vi "Demo.vi"() -> ()   [LabVIEW 2018]
uses:
  api/Log Levels.ctl
  api/Failure Information.ctl
  api/Log Record.ctl
  api/logger_class/Internal Log Levels.ctl
  api/extension/filter_interface/Match Behavior.ctl
  5758470c-db3e-42ca-811c-825e9724b0d9.vi
  30f214a0-5d11-42b7-bf48-9498a62074b5.vi
  4d4d1e0d-ca84-4252-a363-7338c056865d.vi
  e9fdd159-732b-4b71-b39a-13da20540399.vi
  514e4c3d-4430-404b-bd65-5c4555decd7a.vi
  f7cffa30-522c-4f2e-8b3f-df899d765069.vi
  6bf7c309-aeaa-44f2-9fe0-d02c6e1e6f2a.vi
  b04b80c8-7d4a-4373-a7ed-4e6fc68618ba.vi
  82079a54-0ade-4b6d-97e0-3412ec680245.vi
  28c04e52-e175-4a95-b6fe-3645044e5316.vi
  f0baf2eb-a7d9-4d62-b153-bba25fce558d.vi
  f6dcc986-d3e7-4001-b7d2-0cb11a3872ca.vi
  8dbb979e-3c8b-43bd-9788-6e6dcdfca317.vi
  5758470c-db3e-42ca-811c-825e9724b0d9.vi/caf2d4a3-5a7b-40e1-b7b0-74b52901b9f9.vi
  30f214a0-5d11-42b7-bf48-9498a62074b5.vi/bf655d3c-1ce4-400f-a78f-0f3f0191886e.vi
  api/Mark Error.vi
  4d4d1e0d-ca84-4252-a363-7338c056865d.vi/bf655d3c-1ce4-400f-a78f-0f3f0191886e.vi
  e9fdd159-732b-4b71-b39a-13da20540399.vi/ba94d47b-0e30-4c32-b8ff-86d609cd95a5.vi
  514e4c3d-4430-404b-bd65-5c4555decd7a.vi/ba94d47b-0e30-4c32-b8ff-86d609cd95a5.vi
  f7cffa30-522c-4f2e-8b3f-df899d765069.vi/de1063af-56d8-4a46-86b0-d7db6137800f.vi
  6bf7c309-aeaa-44f2-9fe0-d02c6e1e6f2a.vi/de1063af-56d8-4a46-86b0-d7db6137800f.vi
  b04b80c8-7d4a-4373-a7ed-4e6fc68618ba.vi/6f202c45-f0ca-42f4-9f63-a87d9fe0c32d.vi
  82079a54-0ade-4b6d-97e0-3412ec680245.vi/73f0ec31-6bdf-4568-9d3b-fef50ac01b30.vi
  28c04e52-e175-4a95-b6fe-3645044e5316.vi/0a1ee2ab-da6d-4243-8cf3-8125e611a602.vi
  5758470c-db3e-42ca-811c-825e9724b0d9.vi/caf2d4a3-5a7b-40e1-b7b0-74b52901b9f9.vi/0a1ee2ab-da6d-4243-8cf3-8125e611a602.vi
  api/configuration/scopes/basic_scope/Basic.lvclass
  C:/Users/Colin/Documents/software_projects/labview/glog/src/api/extension/scope_interface/Scope.lvclass
  api/configuration/formatters/format_string_formatter/Format String.lvclass
  C:/Users/Colin/Documents/software_projects/labview/glog/src/api/extension/formatter_interface/Formatter.lvclass
  api/configuration/handlers/string_handler/String Handler.lvclass
  C:/Users/Colin/Documents/software_projects/labview/glog/src/api/extension/formatting_handler_interface/Formatting Handler.lvclass
  api/configuration/handlers/file_handler/File Handler.lvclass
  api/configuration/scopes/basic_scope/New (Element).vi
  registry/Log.vi
  <vilib>/Utility/error.llb/Error Cluster From Error Code.vi
  registry/Enable All.vi
  registry/Disable All.vi
  <vilib>/ErrorRing/Error Ring.xnode
  api/GLog.lvlib
panel:
  in  "format string":T1(ring)
  in  "include descendants?":bool caption="Include Descendants?"
  in  "match behavior":T2
  in  "scope":enum16{"Demo", "SubVI", "SubSubVI"}(ring)
  in  "call tree loop":bool caption="Enable Loop"
  in  "error loop":bool caption="Enable Loop"
  in  "basic loop":bool caption="Enable Loop"
  out "log directory":path
  in  "log delay [ms]":i32=100
  in  "log files":i32(listbox)
  in  "error":bool
  in  "warn":bool
  out "failures info":T3[](array[typedef]) {"Log Record"."timestamp" format="%<%x %.3X>T"}
  out "error out":errorcluster
  in  "set lvl all":bool
  in  "disable all":bool
  in  "enable all":bool
  in  "set lvl":bool
  in  "log level":T6
  in  "Loggers":i32(listbox)
  in  "Quit":bool
  out "string logs":string
  in  "disable":bool
  in  "enable":bool
  # "State Control"
  # "Log Level Control"
  # "Speed"
  # "Generic Logging"
  # "Errors/Warnings"
  # "SubVIs"
  # "%^<%Y-%m-%dT%H:%M:%S%3uZ>T | %8L | %M"
  # "%<%a, %b %d, %Y | %I:%M %p>T | %8L | %M"
  # "%<%I:%M:%S %p>T | %8L | %M"
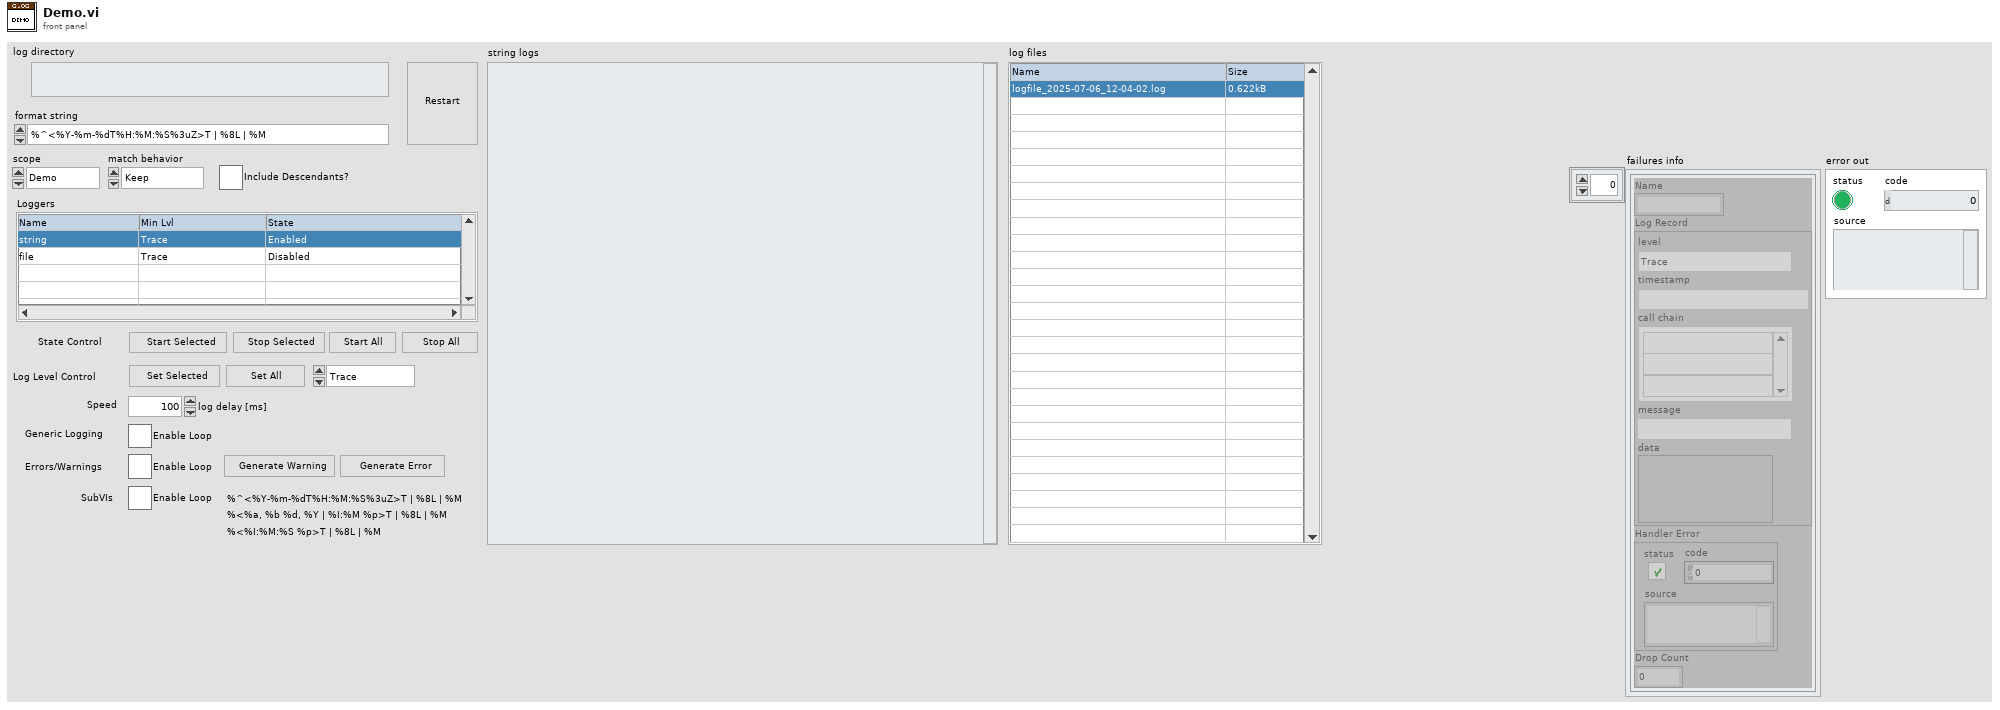
[diagram p1: front panel]
types:
  T1 = enum16{"%^<%Y-%m-%dT%H:%M:%S%3uZ>T | %8L | %M", "%<%a, %b %d, %Y | %I:%M %p>T | %8L | %M", "%<%I:%M:%S %p>T | %8L | %M", "%-30M | %C"}
  T2 = typedef "GLog.lvlib/Match Behavior.ctl" = enum16{"Keep", "Discard"}
  T3 = typedef "GLog.lvlib/Failure Information.ctl" = cluster{"Name":string, "Log Record":T4, "Handler Error":errorcluster, "Drop Count":u32}
  T4 = typedef "GLog.lvlib/Log Record.ctl" = cluster{"level":T5, "timestamp":timestamp, "call chain":string[], "message":string, "data":variant}
  T5 = typedef "GLog.lvlib/Internal Log Levels.ctl" = enum16{"Trace", "Debug", "Info", "Warning", "Error", "Critical", "Internal"}
  T6 = typedef "GLog.lvlib/Log Levels.ctl" = enum16{"Trace", "Debug", "Info", "Warning", "Error", "Critical"}
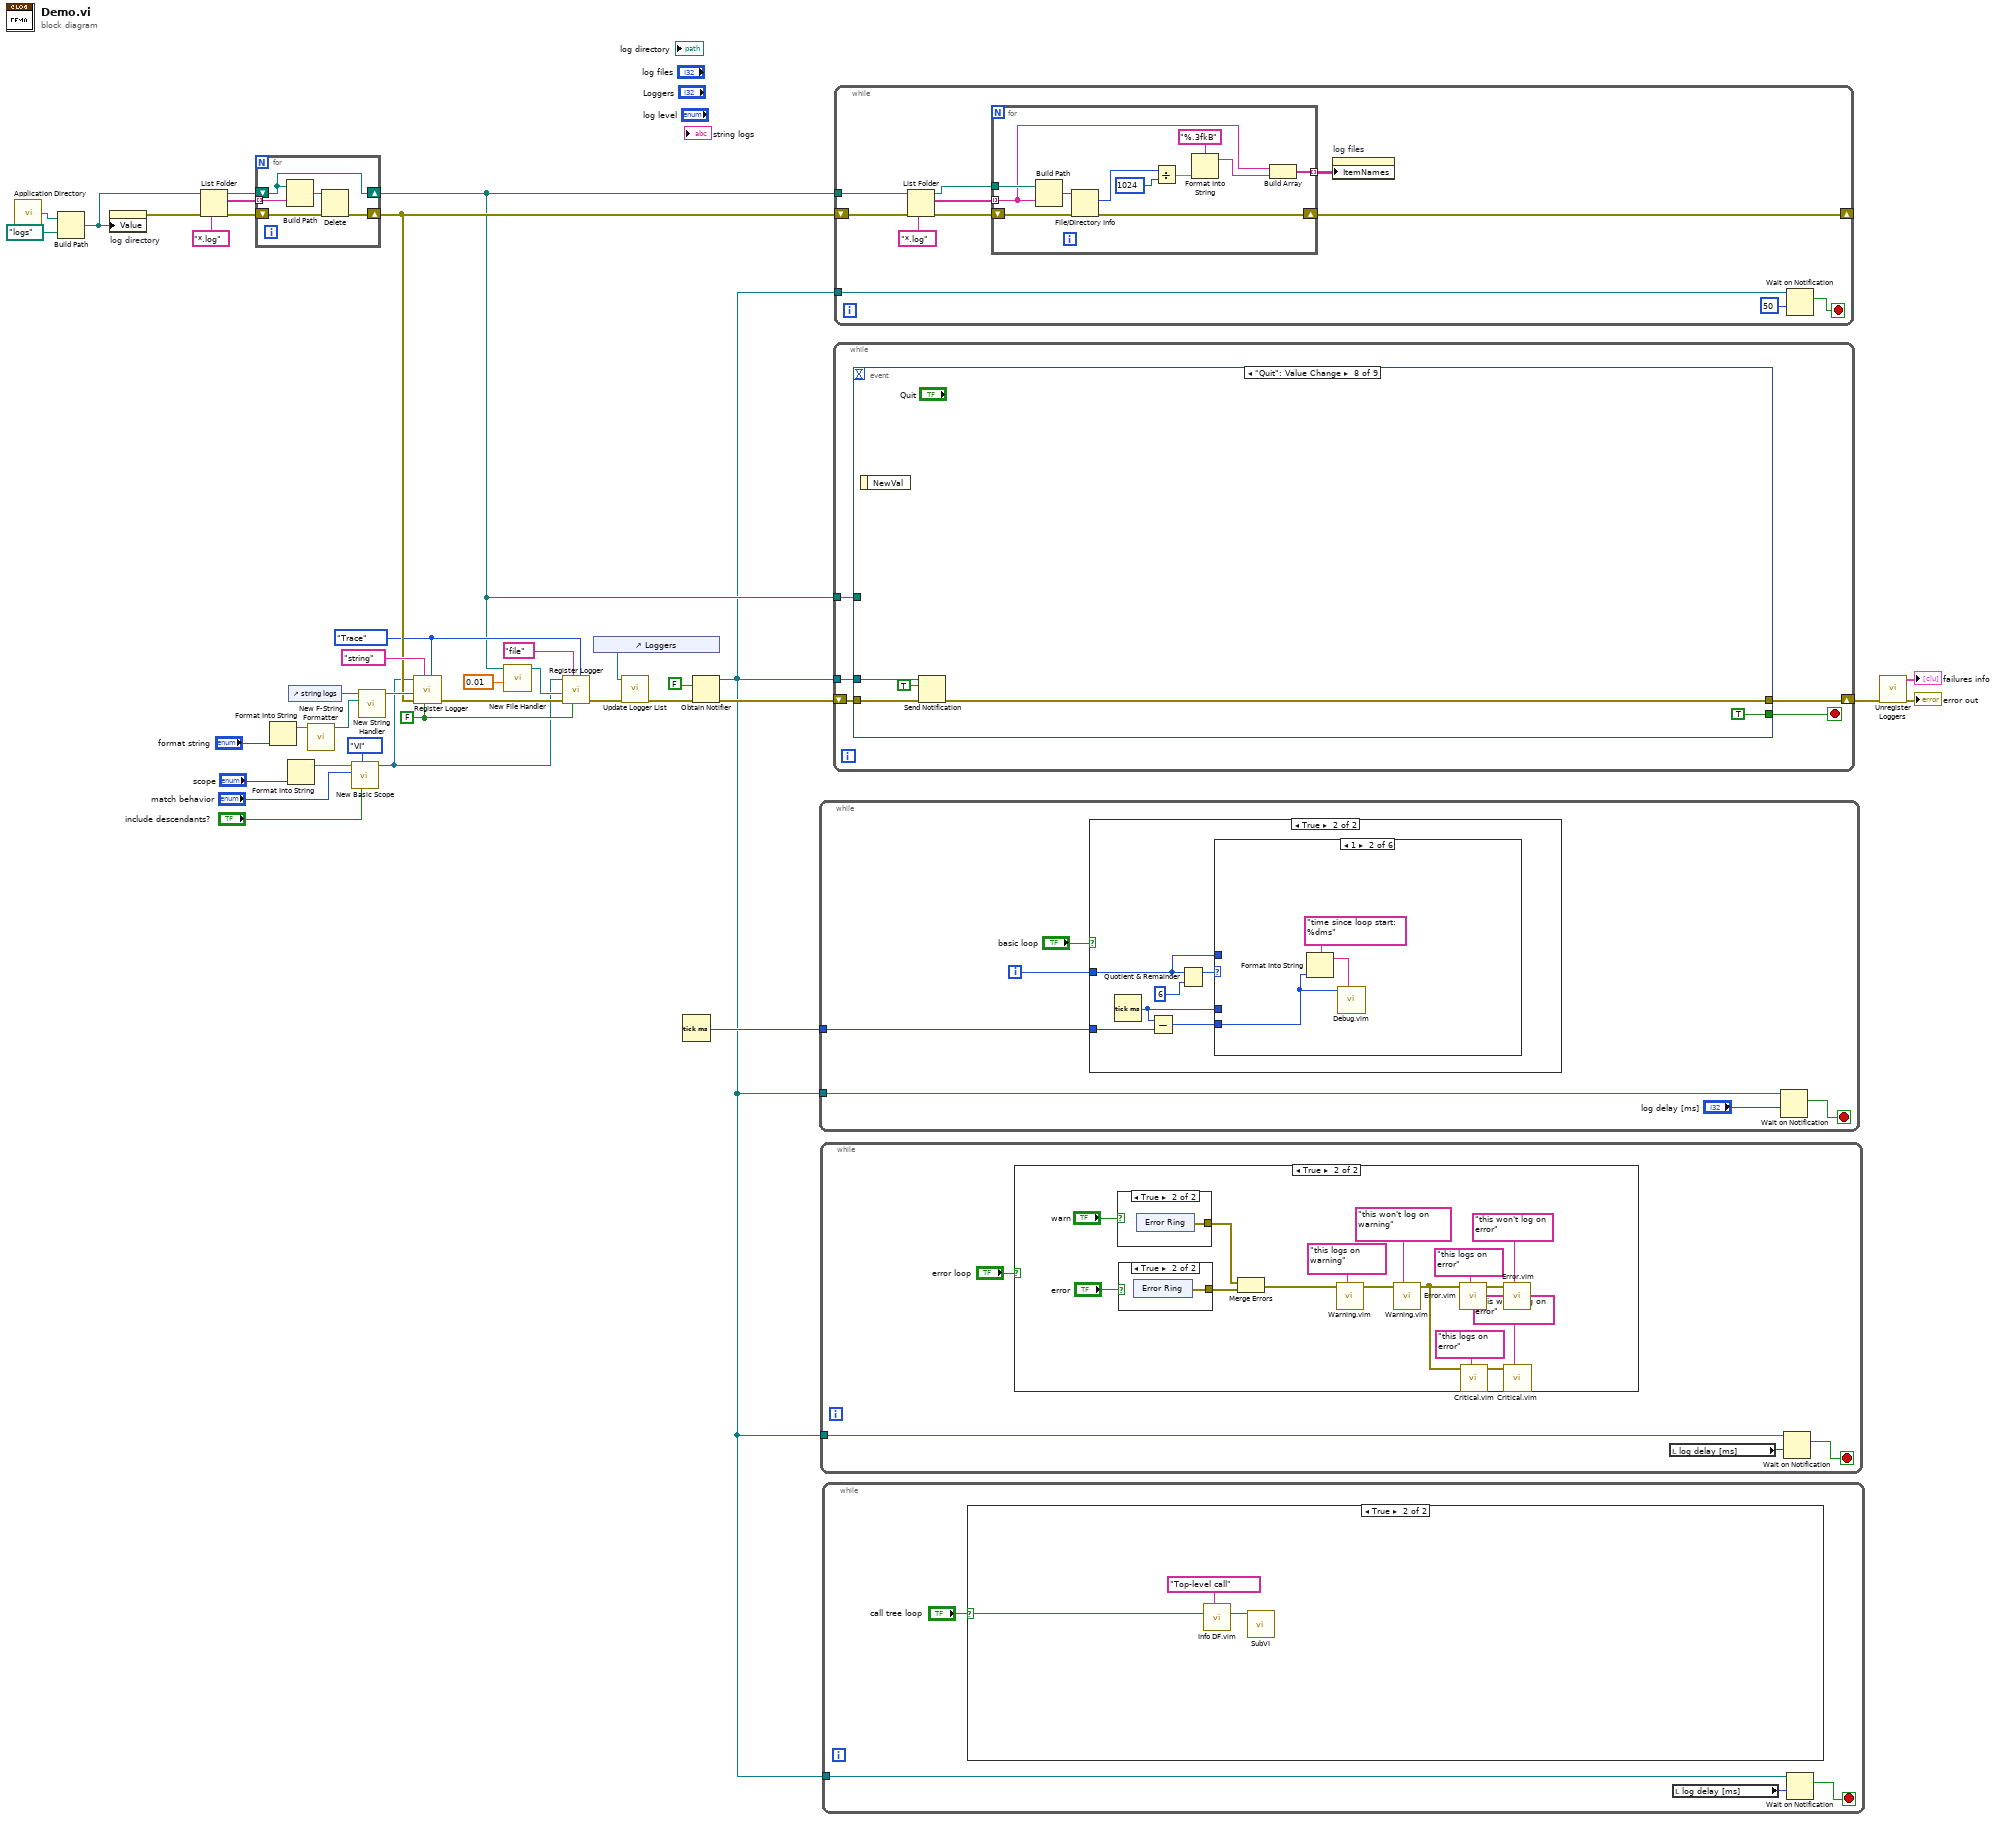
[diagram p0: block diagram]
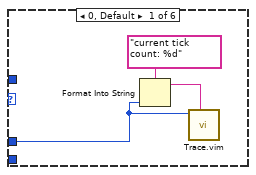
[diagram p7: hidden frame]
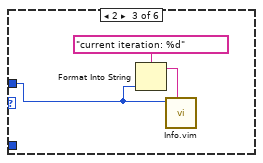
[diagram p8: hidden frame]
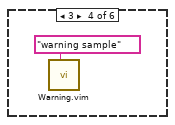
[diagram p9: hidden frame]
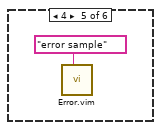
[diagram p10: hidden frame]
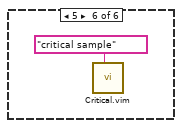
[diagram p11: hidden frame]
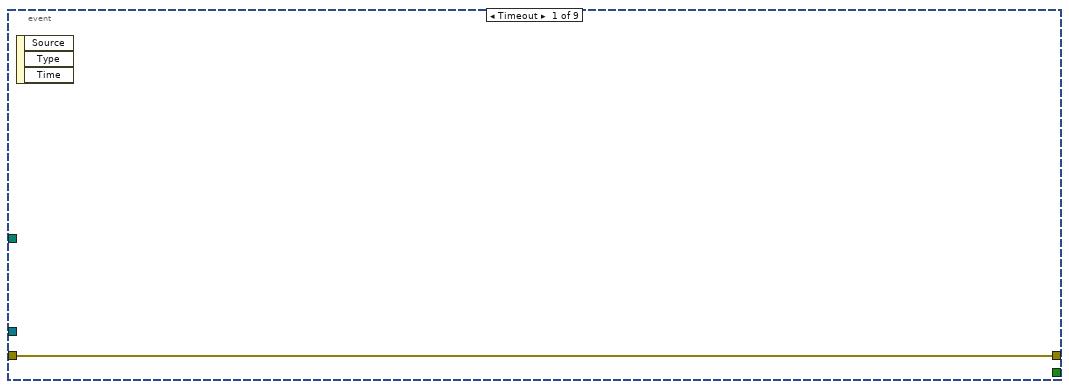
[diagram p12: hidden frame]
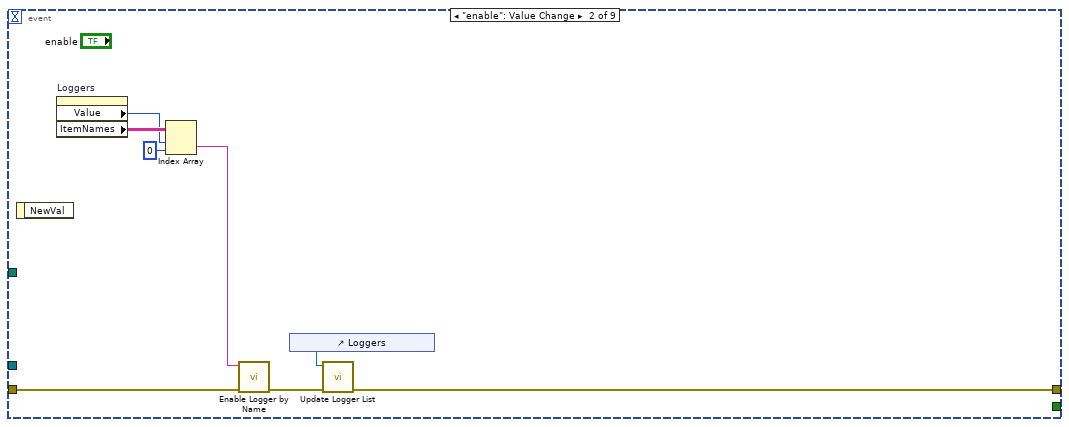
[diagram p13: hidden frame]
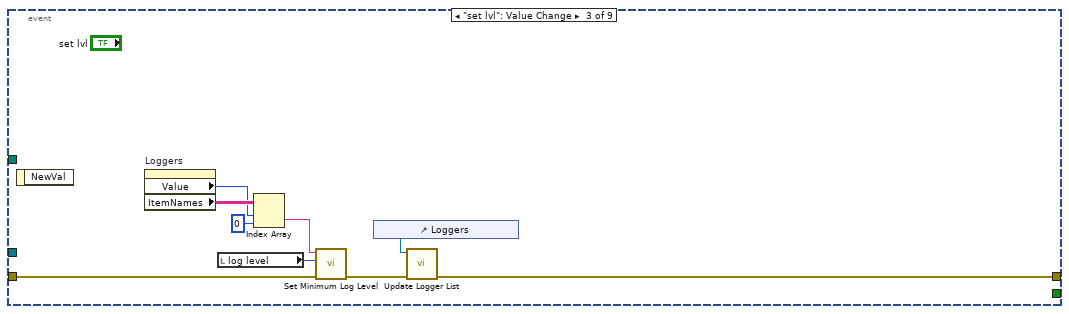
[diagram p14: hidden frame]
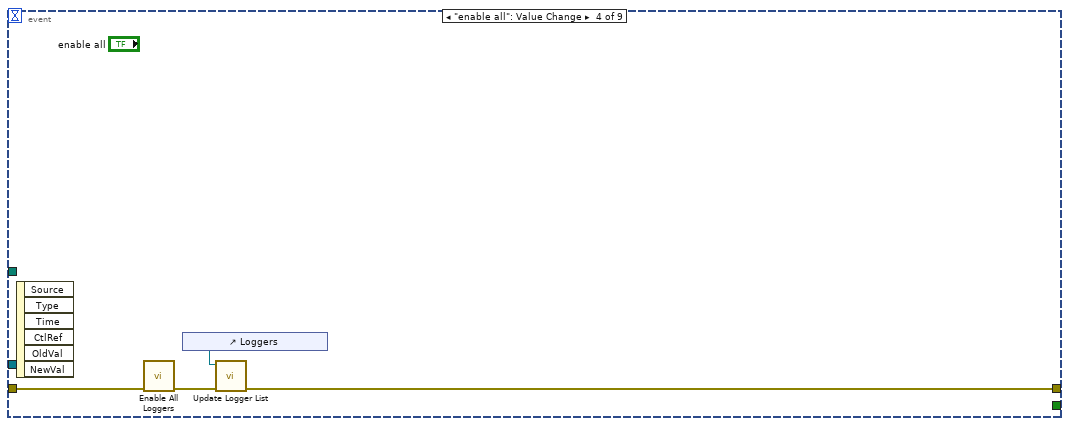
[diagram p15: hidden frame]
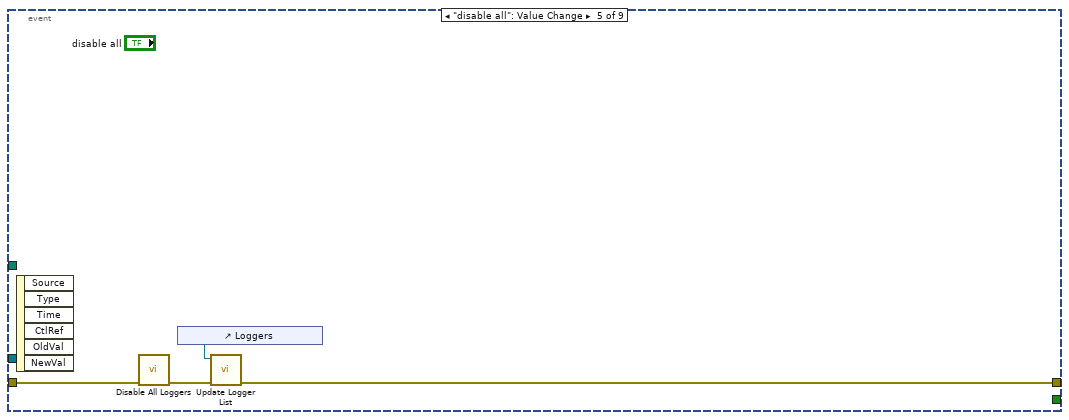
[diagram p16: hidden frame]
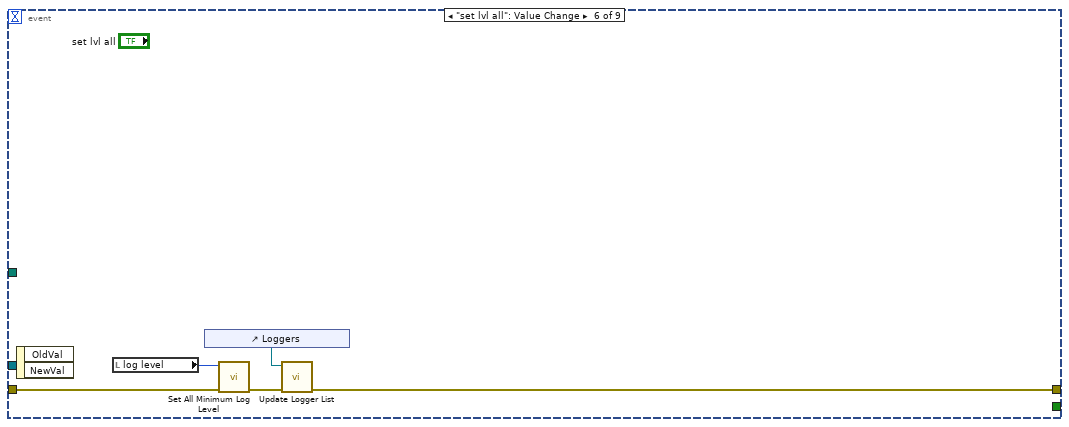
[diagram p17: hidden frame]
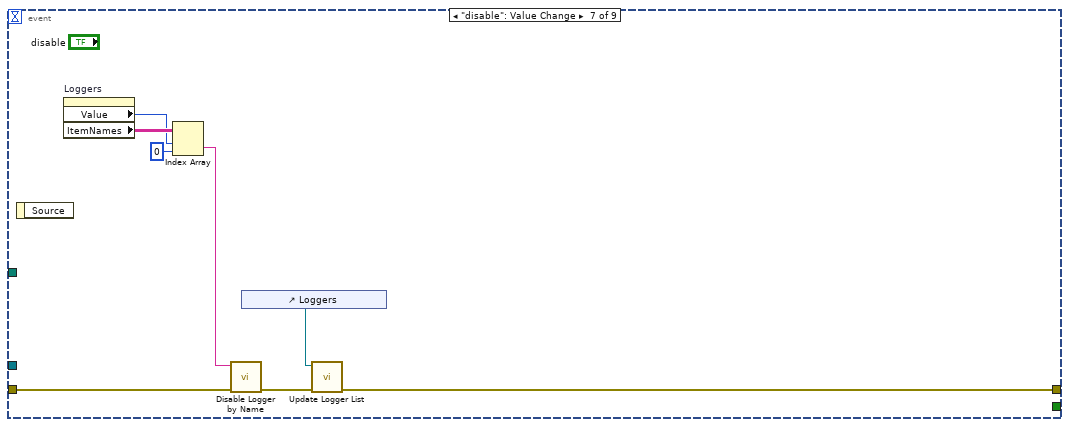
[diagram p18: hidden frame]
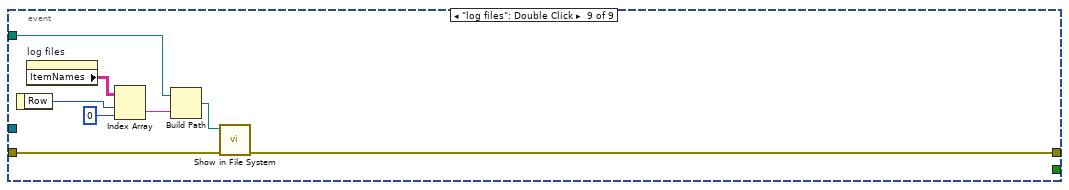
[diagram p19: hidden frame]
diagram:
  w15 = Log_Levels."Trace" ("minimum log level (Info)")
  w35 = FALSE ("enabled? (T)")
  n1 = call <vilib>:"Application Directory.vi"() -> ("Application Directory"=w11:path)
  n2 = Build Path(base path=w11, name or relative path=path "logs") -> (appended path=w12:path)
  n3 = property on="log directory" class="Path"("Value"=w12) -> (error out=w14:errorcluster)  [unwired: 2 in, 1 out]
  n4 = List Folder(path=w12, pattern="*.log", error in=w14) -> (path out=w19:path, filenames=w20:string[], error out=w18:errorcluster)  [unwired: 1 in, 1 out]
  n5 = for {
    tunnel: w20 -> [w43] mode=indexing
    shift-right: [w39] -> w13
    shift-left: w19 -> [w39]
    shift-right: [w40] -> w16
    shift-left: w18 -> [w41]
    n6 = Build Path(base path=w39, name or relative path=w43) -> (appended path=w42:path)
    n7 = Delete(path (use dialog)=w42, error in=w41) -> (error out=w40:errorcluster)  [unwired: 3 in, 2 out]
  }
  n8 = Format Into String("format string") -> (resulting string=w1:string)  [unwired: 3 in, 1 out]
  n9 = Format Into String("scope") -> (resulting string=w6:string)  [unwired: 3 in, 1 out]
  n10 = control-ref of="string logs"() -> (w31:refnum<vi>)
  n11 = call "New F-String Formatter.vi"("format string (\"%T | %L | %M\")"=w1) -> ("new f-string formatter"=w17:refnum<class "Format String.lvclass">)  [unwired: 10 in]
  n12 = call-poly "New Basic Scope.vi"("include descendants? (T)"="include descendants?", "scope type (VI)"=enum16{"VI", "Library", "Class"}."VI", "match behavior (keep)"="match behavior", "scope name (\"\")"=w6) -> ("basic scope"=w3:refnum<class "Basic.lvclass">)  [unwired: 7 in]
  n13 = call "New String Handler.vi"("formatter (format string)"=w17, "string control"=w31) -> ("new string handler"=w32:refnum<class "String Handler.lvclass">)  [unwired: 9 in]
  n14 = call "Register Logger.vi"("minimum log level (Info)"=w15, "enabled? (T)"=w35, "name (\"Default\")"="string" ("name (\"Default\")"), "error in (no error)"=w16, "log handler (file handler)"=w32, "logger scope (all)"=w3) -> ("error out"=w38:errorcluster)  [unwired: 5 in]
  n15 = call "New File Handler.vi"("rollover threshold [MB](50)"=0.01, "log directory (<app dir>/logs)"=w13) -> ("file handler"=w23:refnum<class "File Handler.lvclass">)  [unwired: 9 in]
  n16 = call "Register Logger.vi"("minimum log level (Info)"=w15, "enabled? (T)"=w35, "name (\"Default\")"="file" ("name (\"Default\")"), "error in (no error)"=w38, "log handler (file handler)"=w23, "logger scope (all)"=w3) -> ("error out"=w33:errorcluster)  [unwired: 5 in]
  n17 = control-ref of="Loggers"() -> (w34:refnum<vi>)
  n18 = call "Update Logger List.vi"("error in (no error)"=w33, "MulticolumnListbox in"=w34) -> ("error out"=w27:errorcluster)  [unwired: 9 in]
  n19 = Tick Count (ms)() -> (millisecond timer value=w24:u32)
  n20 = Obtain Notifier(notification data type=FALSE, error in (no error)=w27) -> (notifier out=w9:refnum<notifier>, error out=w26:errorcluster)  [unwired: 2 in, 1 out]
  n21 = while {
    tunnel: w9 -> [w48]
    tunnel: w24 -> [w47]
    i -> [w46]
    stop <- w49 stop-if-true
    n22 = case shown="True" "basic loop" {
      tunnel: w47 -> [_ w53]
      tunnel: w46 -> [_ w52]
      frame False {
      }
      frame True {
        n23 = Tick Count (ms)() -> (millisecond timer value=w50:u32)
        n24 = Subtract(x=w50, y=w53) -> (x-y=w51:u32)
        n25 = Quotient & Remainder(x=w52, y=6) -> (x-y*floor(x/y)=w54:i32)  [unwired: 1 out]
        n26 = case shown="1" w54 {
          tunnel: w52 -> [_ _ w62 _ _ _]
          tunnel: w51 -> [_ w61 _ _ _ _]
          tunnel: w50 -> [w58 _ _ _ _ _]
          frame 0, Default {
            n27 = Format Into String(format string="current tick count: %d" ("message"), w58) -> (resulting string=w57:string)  [unwired: 2 in, 1 out]
            n28 = call "Trace.vim"("data in (null)"=w58, "message"=w57) -> ()  [unwired: 9 in, 1 out]
          }
          frame 1 {
            n29 = Format Into String(format string="time since loop start: %dms" ("message"), w61) -> (resulting string=w59:string)  [unwired: 2 in, 1 out]
            n30 = call "Debug.vim"("data in (null)"=w61, "message"=w59) -> ()  [unwired: 9 in, 1 out]
          }
          frame 2 {
            n31 = Format Into String(format string="current iteration: %d" ("message"), w62) -> (resulting string=w63:string)  [unwired: 2 in, 1 out]
            n32 = call "Info.vim"("data in (null)"=w62, "message"=w63) -> ()  [unwired: 9 in, 1 out]
          }
          frame 3 {
            n33 = call "Warning.vim"("message"="warning sample") -> ()  [unwired: 10 in, 1 out]
          }
          frame 4 {
            n34 = call "Error.vim"("message"="error sample") -> ()  [unwired: 10 in, 1 out]
          }
          frame 5 {
            n35 = call "Critical.vim"("message"="critical sample") -> ()  [unwired: 10 in, 1 out]
          }
        }
      }
    }
    n36 = Wait on Notification(notifier=w48, timeout in ms (-1)="log delay [ms]") -> (notification=w49:bool)  [unwired: 2 in, 3 out]
  }
  n37 = while {
    tunnel: w9 -> [w70]
    stop <- w71 stop-if-true
    n38 = case shown="True" "error loop" {
      frame False {
      }
      frame True {
        n39 = case shown="True" "warn" {
          tunnel: [_ w93] -> w85
          frame False {
          }
          frame True {
            n40 = xnode "Error Ring"() -> ("error out"=w93:errorcluster)
          }
        }
        n41 = case shown="True" "error" {
          tunnel: [_ w87] -> w86
          frame False {
          }
          frame True {
            n42 = xnode "Error Ring"() -> ("error out"=w87:errorcluster)
          }
        }
        n43 = Merge Errors(w85, w86) -> (w73:errorcluster)
        n44 = call "Warning.vim"("data in (null)"=w73, "message"="this logs on warning") -> ("data out"=w80:errorcluster)  [unwired: 9 in]
        n45 = call "Warning.vim"("data in (null)"=w80, "message"="this won't log on warning") -> ("data out"=w72:errorcluster)  [unwired: 9 in]
        n46 = call "Error.vim"("data in (null)"=w72, "message"="this logs on error") -> ("data out"=w77:errorcluster)  [unwired: 9 in]
        n47 = call "Critical.vim"("data in (null)"=w72, "message"="this logs on error") -> ("data out"=w74:errorcluster)  [unwired: 9 in]
        n48 = call "Error.vim"("data in (null)"=w77, "message"="this won't log on error") -> ()  [unwired: 9 in, 1 out]
        n49 = call "Critical.vim"("data in (null)"=w74, "message"="this won't log on error") -> ()  [unwired: 9 in, 1 out]
      }
    }
    n50 = local read "log delay [ms]"() -> (w69:i32)
    n51 = Wait on Notification(notifier=w70, timeout in ms (-1)=w69) -> (notification=w71:bool)  [unwired: 2 in, 3 out]
  }
  n52 = while {
    tunnel: w9 -> [w101]
    stop <- w102 stop-if-true
    n53 = case shown="True" "call tree loop" {
      selector: "call tree loop" -> [_ w104]
      frame False {
      }
      frame True {
        n54 = call "Info DF.vim"("message"="Top-level call", "dataflow in"=w104) -> ("dataflow out"=w103:bool)  [unwired: 9 in]
        n55 = call "SubVI.vi"("dataflow in"=w103) -> ()  [unwired: 11 in]
      }
    }
    n56 = local read "log delay [ms]"() -> (w100:i32)
    n57 = Wait on Notification(notifier=w101, timeout in ms (-1)=w100) -> (notification=w102:bool)  [unwired: 2 in, 3 out]
  }
  n58 = while {
    shift-right: [w109] -> w30
    shift-left: w26 -> [w110]
    tunnel: w9 -> [w108]
    tunnel: w13 -> [w107]
    stop <- w106 stop-if-true
    n59 = event shown="[7] \"Quit\": Value Change" {
      selector: _ -> [_ _ _ _ _ _ _ _ _]
      dyn-events: _ -> [_ _ _ _ _ _ _ _ _]
      timeout: _ -> [_ _ _ _ _ _ _ _ _]
      tunnel: [_ _ _ _ _ _ _ TRUE _] -> w106
      tunnel: [w111 w112 w120 w129 w134 w139 w143 w153 w156] -> w109
      tunnel: w110 -> [w111 w115 w128 w132 w133 w138 w145 w152 w155]
      tunnel: w108 -> [_ _ _ _ _ _ _ w151 _]
      tunnel: w107 -> [_ _ _ _ _ _ _ _ w158]
      event Timeout {
        n60 = event-data() -> ()  [unwired: 1 in, 3 out]
      }
      event "enable": Value Change {
        n61 = event-data() -> ()  [unwired: 1 in, 1 out]
        n62 = property on="Loggers" class="MCListbox (strict)"() -> ("Value"=w118:i32, "ItemNames"=w119:string[][])  [unwired: 2 in, 2 out]
        n63 = Index Array(array=w119, index (row)=w118, index (col)=0 ("disabled index (col)")) -> (element=w116:string)
        n64 = call "Enable Logger by Name.vi"("error in (no error)"=w115, "name (\"Default\")"=w116) -> ("error out"=w113:errorcluster)  [unwired: 9 in]
        n65 = control-ref of="Loggers"() -> (w114:refnum<vi>)
        n66 = call "Update Logger List.vi"("error in (no error)"=w113, "MulticolumnListbox in"=w114) -> ("error out"=w112:errorcluster)  [unwired: 9 in]
      }
      event "set lvl": Value Change {
        n67 = event-data() -> ()  [unwired: 1 in, 1 out]
        n68 = property on="Loggers" class="MCListbox (strict)"() -> ("Value"=w125:i32, "ItemNames"=w126:string[][])  [unwired: 2 in, 2 out]
        n69 = local read "log level"() -> (w127:T6)
        n70 = Index Array(array=w126, index (row)=w125, index (col)=0 ("disabled index (col)")) -> (element=w123:string)
        n71 = call "Set Minimum Log Level.vi"("error in (no error)"=w128, "log level (Info)"=w127, "name (\"Default\")"=w123) -> ("error out"=w121:errorcluster)  [unwired: 8 in]
        n72 = control-ref of="Loggers"() -> (w122:refnum<vi>)
        n73 = call "Update Logger List.vi"("error in (no error)"=w121, "MulticolumnListbox in"=w122) -> ("error out"=w120:errorcluster)  [unwired: 9 in]
      }
      event "enable all": Value Change {
        n74 = event-data() -> ()  [unwired: 1 in, 6 out]
        n75 = call "Enable All Loggers.vi"("error in"=w132) -> ("error out"=w130:errorcluster)  [unwired: 10 in]
        n76 = control-ref of="Loggers"() -> (w131:refnum<vi>)
        n77 = call "Update Logger List.vi"("error in (no error)"=w130, "MulticolumnListbox in"=w131) -> ("error out"=w129:errorcluster)  [unwired: 9 in]
      }
      event "disable all": Value Change {
        n78 = event-data() -> ()  [unwired: 1 in, 6 out]
        n79 = call "Disable All Loggers.vi"("error in"=w133) -> ("error out"=w135:errorcluster)  [unwired: 10 in]
        n80 = control-ref of="Loggers"() -> (w136:refnum<vi>)
        n81 = call "Update Logger List.vi"("error in (no error)"=w135, "MulticolumnListbox in"=w136) -> ("error out"=w134:errorcluster)  [unwired: 9 in]
      }
      event "set lvl all": Value Change {
        n82 = event-data() -> ()  [unwired: 1 in, 2 out]
        n83 = local read "log level"() -> (w137:T6)
        n84 = control-ref of="Loggers"() -> (w141:refnum<vi>)
        n85 = call "Set All Minimum Log Level.vi"("error in"=w138, "log level (Info)"=w137) -> ("error out"=w140:errorcluster)  [unwired: 9 in]
        n86 = call "Update Logger List.vi"("error in (no error)"=w140, "MulticolumnListbox in"=w141) -> ("error out"=w139:errorcluster)  [unwired: 9 in]
      }
      event "disable": Value Change {
        n87 = event-data() -> ()  [unwired: 1 in, 1 out]
        n88 = property on="Loggers" class="MCListbox (strict)"() -> ("Value"=w148:i32, "ItemNames"=w149:string[][])  [unwired: 2 in, 2 out]
        n89 = Index Array(array=w149, index (row)=w148, index (col)=0 ("disabled index (col)")) -> (element=w147:string)
        n90 = call "Disable Logger by Name.vi"("error in (no error)"=w145, "name (\"Default\")"=w147) -> ("error out"=w144:errorcluster)  [unwired: 9 in]
        n91 = control-ref of="Loggers"() -> (w142:refnum<vi>)
        n92 = call "Update Logger List.vi"("error in (no error)"=w144, "MulticolumnListbox in"=w142) -> ("error out"=w143:errorcluster)  [unwired: 9 in]
      }
      event "Quit": Value Change {
        n93 = event-data() -> ()  [unwired: 1 in, 1 out]
        n94 = Send Notification(notification=TRUE, notifier=w151, error in (no error)=w152) -> (error out=w153:errorcluster)  [unwired: 1 out]
      }
      event "log files": Double Click {
        n95 = event-data() -> ("Row"=w161:i32)  [unwired: 1 in]
        n96 = property on="log files" class="MCListbox (strict)"() -> ("ItemNames"=w162:string[][])  [unwired: 2 in, 2 out]
        n97 = Index Array(array=w162, index (row)=w161, index (col)=0 ("disabled index (col)")) -> (element=w159:string)
        n98 = Build Path(base path=w158, name or relative path=w159) -> (appended path=w157:path)
        n99 = call <vilib>:"Show in File System.vi"("error in (no error)"=w155, "file or directory path"=w157) -> ("error out"=w156:errorcluster)  [unwired: 9 in]
      }
    }
  }
  n100 = while {
    tunnel: w13 -> [w173]
    tunnel: w9 -> [w167]
    shift-right: [w164] -> _
    shift-left: w16 -> [w165]
    stop <- w166 stop-if-true
    n101 = List Folder(path=w173, pattern="*.log", error in=w165) -> (path out=w170:path, filenames=w169:string[], error out=w171:errorcluster)  [unwired: 1 in, 1 out]
    n102 = for {
      tunnel: w170 -> [w183]
      tunnel: w169 -> [w176] mode=indexing
      tunnel: [w174] -> w163 mode=indexing
      shift-right: [w178] -> w164
      shift-left: w171 -> [w184]
      n103 = Build Path(base path=w183, name or relative path=w176) -> (appended path=w182:path)
      n104 = File/Directory Info(path=w182, error in=w184) -> (size=w181:i64, error out=w178:errorcluster)  [unwired: 5 out]
      n105 = Divide(x=w181, y=i64 1024) -> (x/y=w180:dbl)
      n106 = Format Into String(format string="%.3fkB", w180) -> (resulting string=w175:string)  [unwired: 2 in, 1 out]
      n107 = Build Array(w176, w175) -> (w174:string[])
    }
    n108 = property on="log files" class="MCListbox (strict)"("ItemNames"=w163) -> ()  [unwired: 2 in, 2 out]
    n109 = Wait on Notification(notifier=w167, timeout in ms (-1)=50) -> (notification=w166:bool)  [unwired: 2 in, 3 out]
  }
  n110 = call "Unregister Loggers.vi"("error in (no error)"=w30) -> ("error out"=→"error out":errorcluster, "failures info"=→"failures info":T3[])  [unwired: 9 in]
